vi "Lex Text-EndSection-Text.vi"(8 "Error In":errorcluster) -> (0 "Error Out":errorcluster)   [LabVIEW 2018, in "Tests.lvlib" / "Lexer.lvlib"]
uses:
  Lexer.lvlib
  src/Toolkit/Low-Level/Tokens/Text/Text.lvclass
  src/Toolkit/Low-Level/Tokens/EndSection/EndSection.lvclass
  <vilib>/addons/_JKI Toolkits/Caraya/classes/Assert/Assert Equal Type_Variant.vi
  src/Toolkit/Low-Level/Tokens/Contentable/Contentable.lvclass
  src/Toolkit/Low-Level/Tokens/Keyable/Keyable.lvclass
  src/Toolkit/Low-Level/Lexer/Lexer.lvclass
  <vilib>/addons/_JKI Toolkits/Caraya/classes/Test/Test.lvclass
  <vilib>/addons/_JKI Toolkits/Caraya/classes/Assert/Assert.lvclass
  src/Toolkit/Low-Level/Tokens/Token/Token.lvclass
  Tests.lvlib
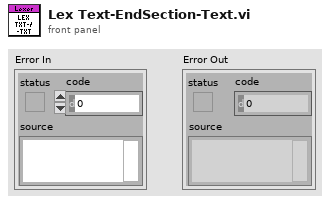
[diagram p1: front panel]
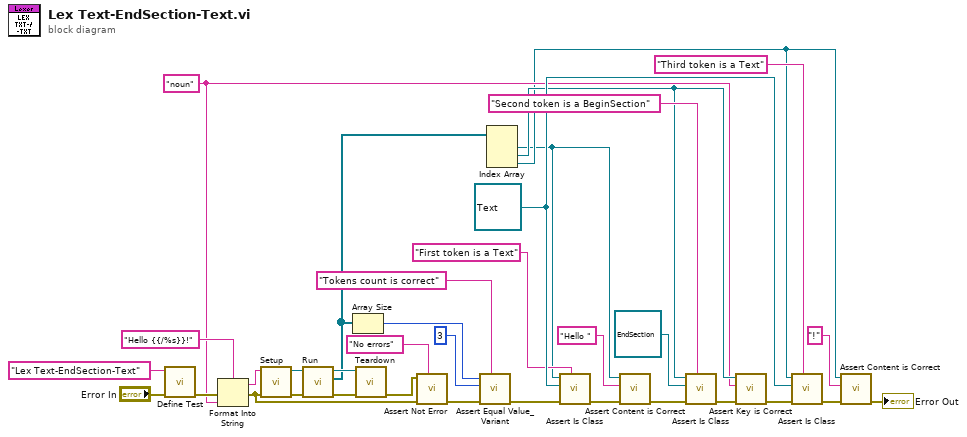
[diagram p0: block diagram]
diagram:
  w20 = refnum<class "Text.lvclass"> refnum ("Mustache.lvlib:Tokens.lvlib:Text.lvclass")
  w14 = "noun" ("String")
  n1 = call <vilib>:"Define Test.vi"("error in (no error)"="Error In", "Label (VI Title)"="Lex Text-EndSection-Text") -> ("error out"=w33:errorcluster)  [unwired: 9 in]
  n2 = Format Into String(format string="Hello {{/%s}}!", error in=w33, w14) -> (resulting string=w3:string, error out=w4:errorcluster)  [unwired: 1 in]
  n3 = call "Setup.vi"("Error In"=w4, "String"=w3) -> ("Error Out"=w7:errorcluster, "Lexer"=w8:refnum<class "Lexer.lvclass">)  [unwired: 8 in]
  n4 = call-dynamic "Run.vi"("Error In"=w7, "Lexer In"=w8) -> ("Error Out"=w5:errorcluster, "Tokens"=w2:refnum<class "Token.lvclass">[], "Lexer Out"=w6:refnum<class "Lexer.lvclass">)  [unwired: 7 in]
  n5 = Array Size(array=w2) -> (size(s)=w29:i32)
  n6 = call "Teardown.vi"("Error In"=w5, "Lexer"=w6) -> ("Error Out"=w1:errorcluster)  [unwired: 9 in]
  n7 = call <vilib>:"Assert Not Error.vi"("Label"="No errors", "error in (no error)"=w4, "Not Error?"=w1) -> ("error out"=w31:errorcluster)  [unwired: 8 in]
  n8 = call <vilib>:"Assert Equal Value_Variant.vi"("Label"="Tokens count is correct", "error in (no error)"=w31, "Y"=3 ("size(s)"), "X"=w29) -> ("error out"=w27:errorcluster)  [unwired: 7 in]
  n9 = Index Array(array=w2) -> (element #1=w10:refnum<class "Token.lvclass">, element #2=w16:refnum<class "Token.lvclass">, element #3=w12:refnum<class "Token.lvclass">)  [unwired: 3 in]
  n10 = call "Assert Is Class.vi"("Label"="First token is a Text", "Error In"=w27, "Expected"=w20, "Actual"=w10) -> ("Error Out"=w25:errorcluster)  [unwired: 7 in]
  n11 = call "Assert Content is Correct.vi"("Error In"=w25, "Expected"="Hello ", "Token"=w10) -> ("Error Out"=w24:errorcluster)  [unwired: 8 in]
  n12 = call "Assert Is Class.vi"("Label"="Second token is a BeginSection", "Error In"=w24, "Expected"=refnum<class "EndSection.lvclass"> refnum ("Mustache.lvlib:Tokens.lvlib:EndSection.lvclass"), "Actual"=w16) -> ("Error Out"=w15:errorcluster)  [unwired: 7 in]
  n13 = call "Assert Key is Correct.vi"("Error In"=w15, "Expected"=w14, "Token"=w16) -> ("Error Out"=w23:errorcluster)  [unwired: 8 in]
  n14 = call "Assert Is Class.vi"("Label"="Third token is a Text", "Error In"=w23, "Expected"=w20, "Actual"=w12) -> ("Error Out"=w22:errorcluster)  [unwired: 7 in]
  n15 = call "Assert Content is Correct.vi"("Error In"=w22, "Expected"="!", "Token"=w12) -> ("Error Out"=→"Error Out":errorcluster)  [unwired: 8 in]
